vi "6-t-dist.vi"(0 "p_LExp":T1, 5 "t":dbl, 11 "error in":errorcluster caption="err in") -> (2 "R(t)":dbl, 3 "La (t)":dbl, 4 "p_LExp":T1, 6 "t":dbl, 8 "f (t)":dbl, 10 "F (t)":dbl, 15 "error out":errorcluster caption="err out")   [LabVIEW 2010, in "lv_02.lvlib"]
uses:
  lv_02.lvlib
  p_5E6_Lexp.ctl
  p_5E7_LW.ctl
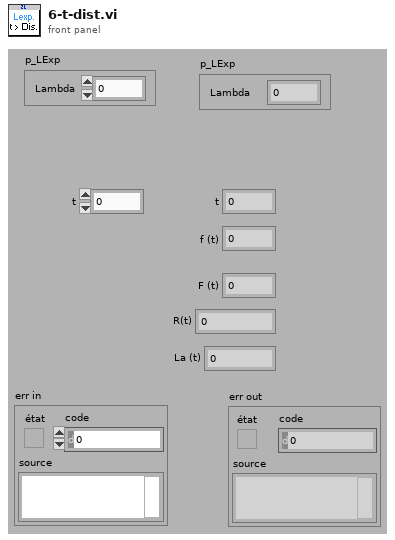
[diagram p1: front panel]
types:
  T1 = typedef "lv_02.lvlib/p_5E6_Lexp.ctl" = cluster{"Lambda":dbl}
  T2 = typedef "lv_02.lvlib/p_5E7_LW.ctl" = cluster{"Beta":dbl, "Eta":dbl, "Gama":dbl}
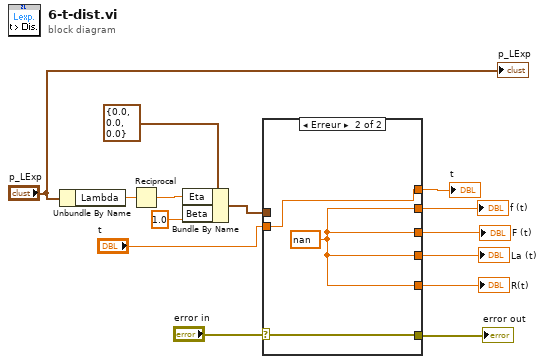
[diagram p0: block diagram]
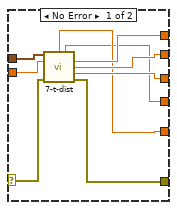
[diagram p2: hidden frame]
diagram:
  n1 = Unbundle By Name("p_LExp") -> ("Lambda"=w5:dbl)
  n2 = Reciprocal(x=w5) -> (1/x=w4:dbl)
  n3 = Bundle By Name(cluster=T2 {"Beta"=0.0, "Eta"=0.0, "Gama"=0.0} ("p_LW"), "Eta"=w4, "Beta"=1.0) -> (w2:T2)
  n4 = case shown="Erreur" "error in" {
    selector: "error in" -> [w21 w26]
    tunnel: "t" -> [w22 w24]
    tunnel: [w15 w25] -> w13
    tunnel: [w20 w26] -> w11
    tunnel: [w17 w25] -> w10
    tunnel: [w16 w25] -> w9
    tunnel: [w18 w25] -> w8
    tunnel: w2 -> [w23 _]
    tunnel: [w19 w24] -> w1
    frame No Error {
      n5 = call "7-t-dist.vi"("p_LW"=w23, "t"=w22, "error in"=w21) -> ("R(t)"=w16:dbl, "La (t)"=w15:dbl, "t"=w19:dbl, "f (t)"=w18:dbl, "F (t)"=w17:dbl, "error out"=w20:errorcluster)  [unwired: 6 in, 1 out]
    }
    frame Error {
      w25 = nan
    }
  }
  "La (t)" <- w13
  "error out" <- w11
  "F (t)" <- w10
  "R(t)" <- w9
  "f (t)" <- w8
  "t" <- w1
  "p_LExp" <- "p_LExp"
